vi "Initialize UI.vi"(6 "menu options":cluster{"open":bool, "save":bool, "view":bool}={"open"=TRUE, "save"=FALSE, "view"=FALSE}, 8 "error in (no error)":errorcluster, 10 "Path":path, 11 "Application Data in":T1) -> (0 "error out":errorcluster, 3 "Application Data out":T1)   [LabVIEW 2017, in "DSF Configuration Utility.lvlib"]
uses:
  DSF Configuration Utility.lvlib
  Application Data.ctl
  VeriStand/Data Sharing Custom Device/Source/Engine/DSF Core.lvlibp/Classes/Configuration/Configuration Session.lvclass
  View Mode.ctl
panel:
  # "App\nData"
  # "App\nData"
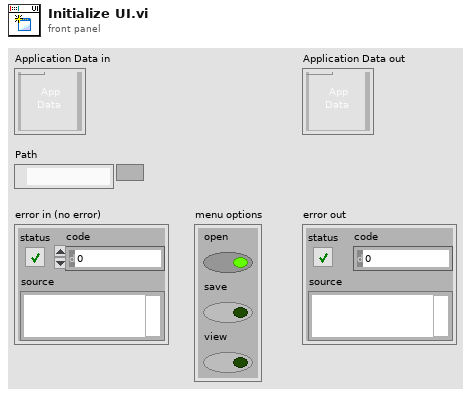
[diagram p1: front panel]
types:
  T1 = typedef "DSF Configuration Utility.lvlib/Application Data.ctl" = cluster{"Item Tree Control":refnum<vi>, "Value Tree Control":refnum<vi>, "DSF Refnum":refnum<class "Configuration Session.lvclass">, "Top-Level VI":refnum<vi>, "View State":T2, "menu reference":refnum<k9>}
  T2 = typedef "DSF Configuration Utility.lvlib/View Mode.ctl" = enum16{"Tree", "List"}
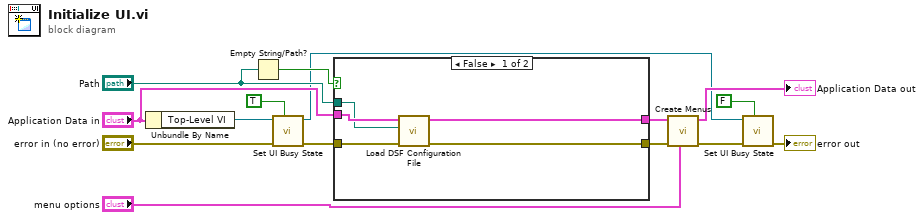
[diagram p0: block diagram]
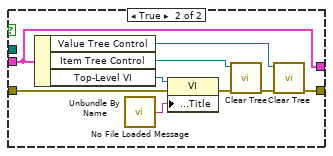
[diagram p2: hidden frame]
diagram:
  n1 = Unbundle By Name("Application Data in") -> ("Top-Level VI"=w4:refnum<vi>)
  n2 = Empty String/Path?(string/path="Path") -> (empty?=w13:bool)
  n3 = call "Set UI Busy State.vi"("Defer Panel Updates"=TRUE, "error in (no error)"="error in (no error)", "VI in"=w4) -> ("error out"=w7:errorcluster, "VI out"=w3:refnum<vi>)  [unwired: 7 in]
  n4 = case shown="False" w13 {
    tunnel: "Path" -> [w17 _]
    tunnel: [w16 w22] -> w14
    tunnel: [w20 w28] -> w10
    tunnel: "Application Data in" -> [w19 w28]
    tunnel: w7 -> [w18 w29]
    frame False {
      n5 = call "Load DSF Configuration File.vi"("error in (no error)"=w18, "Path"=w17, "Application Refs"=w19) -> ("error out"=w16:errorcluster, "Application Data out"=w20:T1)  [unwired: 7 in]
    }
    frame True {
      n6 = Unbundle By Name(w28) -> ("Value Tree Control"=w21:refnum<vi>, "Item Tree Control"=w27:refnum<vi>, "Top-Level VI"=w25:refnum<vi>)
      n7 = call "No File Loaded Message.vi"() -> ("no file loaded string"=w24:string)  [unwired: 1 in]
      n8 = property class="VI"(reference=w25, error in=w29, "Front Panel.Title"=w24) -> (error out=w26:errorcluster)  [unwired: 1 out]
      n9 = call "Clear Tree.vi"("error in (no error)"=w26, "TreeControl in"=w27) -> ("error out"=w23:errorcluster)  [unwired: 9 in]
      n10 = call "Clear Tree.vi"("error in (no error)"=w23, "TreeControl in"=w21) -> ("error out"=w22:errorcluster)  [unwired: 9 in]
    }
  }
  n11 = call "Create Menus.vi"("menu options"="menu options", "error in (no error)"=w14, "Application Data in"=w10) -> ("error out"=w11:errorcluster, "Application Data out"=→"Application Data out":T1)  [unwired: 7 in]
  n12 = call "Set UI Busy State.vi"("Defer Panel Updates"=FALSE, "error in (no error)"=w11, "VI in"=w3) -> ("error out"=→"error out":errorcluster)  [unwired: 7 in, 1 out]
